vi "Initialize.vi"() -> (0 "Draw Message":refnum<class "Draw Message.lvclass">)   [LabVIEW 2019, in "Draw Messages.lvlib" / "Circle Message.lvclass"]
doc: "Initialize a Circle Message."
uses:
  Circle Message.lvclass
  Draw Message/Draw Message.lvclass
  e:/builds/penguin/labview/branches/2019/dev/dist/examples/Channels/Event Messenger/SubVIs/Draw Messages/Draw Message/Draw Message.lvclass
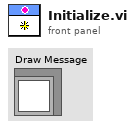
[diagram p1: front panel]
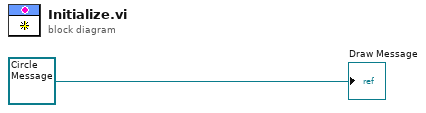
[diagram p0: block diagram]
diagram:
  "Draw Message" <- refnum<class "Circle Message.lvclass"> refnum ("Draw Messages.lvlib:Circle Message.lvclass")
